vi "Select XNET Signals UI.vi"(8 "error in (no error)":errorcluster, 9 "XNET Cluster":refnum<k21>, 10 "XNET Database":refnum<k21>, 11 "Node Ptr":u64 format="%.0x") -> (0 "error out":errorcluster, 2 "Cancel Out":bool, 3 "XNET Signal Names":refnum<k21>[](array[refnum]))   [LabVIEW 2023, in "J1939 Addon System Explorer.lvlib"]
uses:
  J1939 Addon System Explorer.lvlib
  <vilib>/Utility/cursorutil.llb/Set Cursor (Icon Pict).vi
  Addon Shared/J1939 Addon Shared.lvlib
panel:
  in  "Info?":bool
  in  "Cancel":bool
  in  "Select":bool
  in  "Tree":string(tree)
  # "OUTPUTS"
  # "INPUTS"
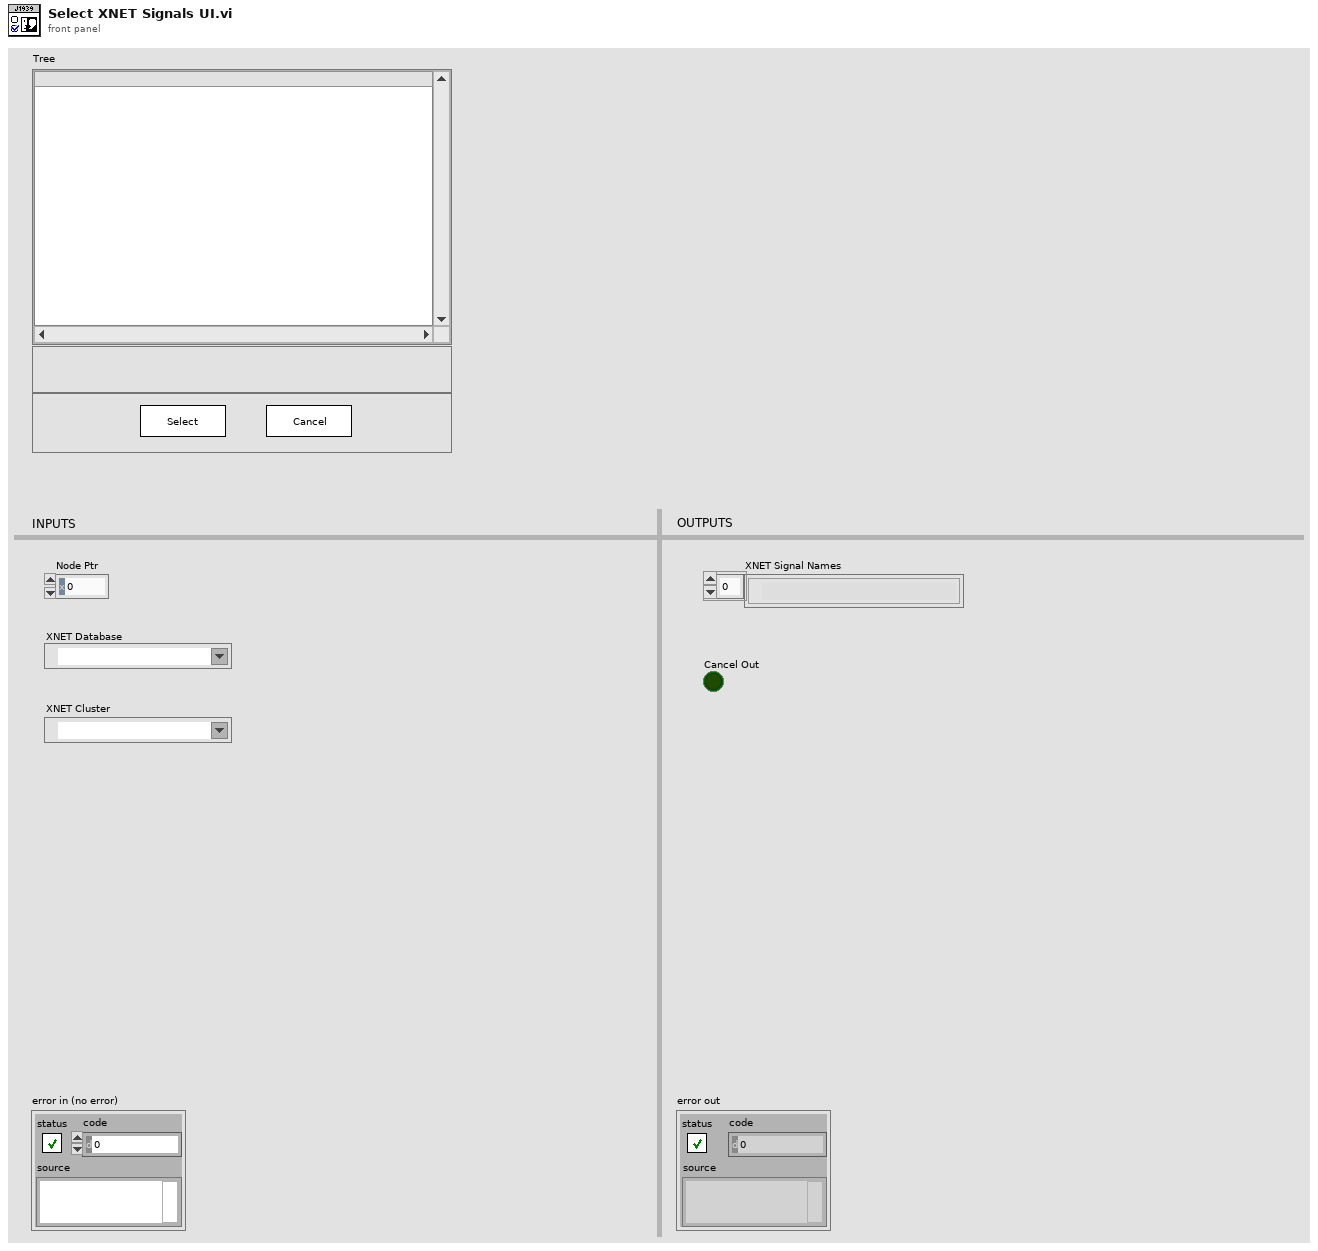
[diagram p1: front panel]
types:
  T1 = typedef "LVPoint32TypeDef.ctl" = cluster{"Horizontal":i32, "Vertical":i32}
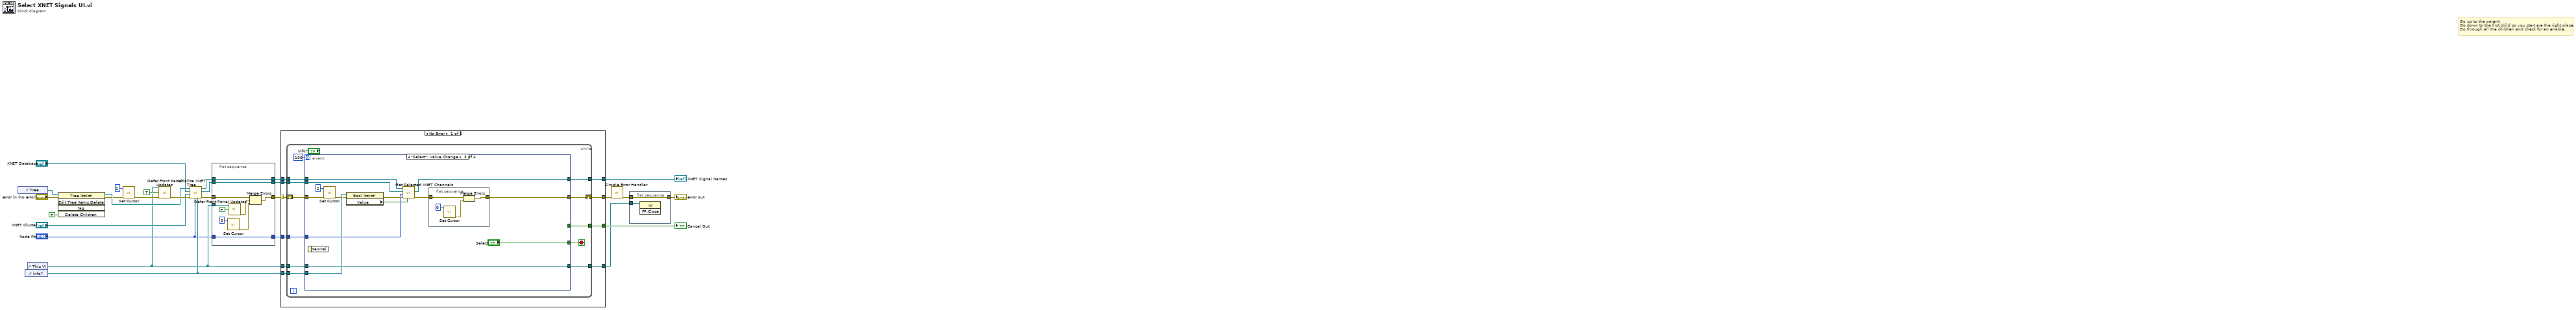
[diagram p0: block diagram]
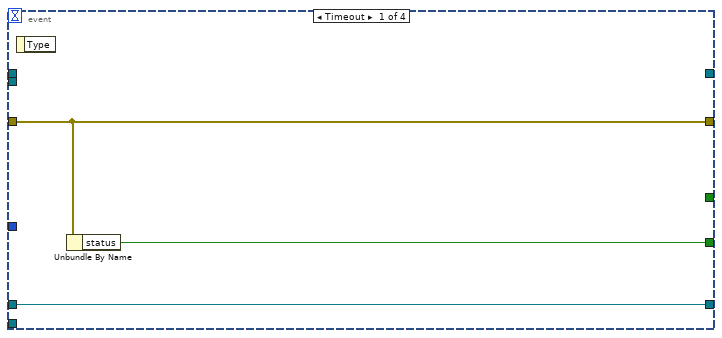
[diagram p2: hidden frame]
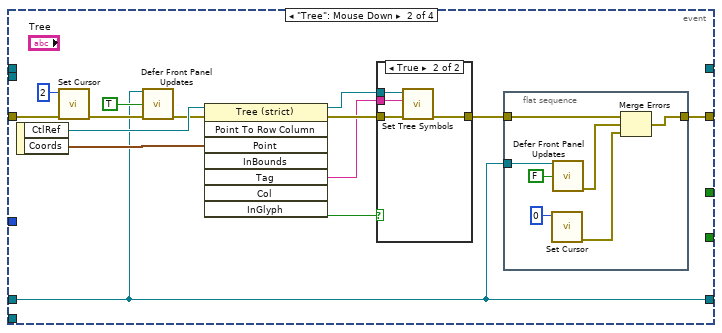
[diagram p3: hidden frame]
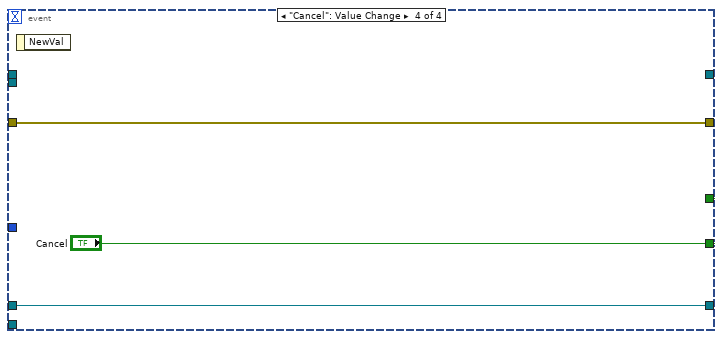
[diagram p5: hidden frame]
diagram:
  # "Go up to the parent.\nGo down to the first child so you start are the right place.\nGo through all the children and check for an enable."
  n1 = control-ref of="Tree"() -> (w14:refnum<vi>)
  n2 = control-ref of="Info?"() -> (w4:refnum<vi>)
  n3 = control-ref of="This VI"() -> (w7:refnum<vi>)
  n4 = invoke on="Invoke Node" class="Tree (strict)" method="Edit Tree Items.Delete"(reference=w14, error in="error in (no error)", "Delete Children"=TRUE ("Delete Children?")) -> (reference out=w13:refnum<vi>, error out=w11:errorcluster)  [unwired: 2 in, 3 out]
  n5 = call-poly <vilib>:"Set Cursor.vi"("error in (no error)"=w11, "icon"=u16 2) -> ("error out"=w10:errorcluster)  [unwired: 8 in, 1 out]
  n6 = call "Defer Front Panel Updates.vi"("This VI"=w7, "Defer Panel Updates"=TRUE, "error in (no error)"=w10) -> ("error out"=w5:errorcluster)  [unwired: 12 in]
  n7 = call "Initialize XNET Tree.vi"("Info?"=w4, "Node Ptr"="Node Ptr", "error in"=w5, "XNET Cluster"="XNET Cluster", "XNET Database"="XNET Database", "Tree"=w13) -> ("error out"=w3:errorcluster, "XNET Cluster Out"=w18:refnum<k21>, "Tree Out"=w1:refnum<vi>)  [unwired: 2 in, 1 out]
  n8 = flat-sequence {
    tunnel: [w36] -> w23
    tunnel: [w33] -> w22
    tunnel: [w31] -> w19
    tunnel: [w30] -> w8
    tunnel: w3 -> [w35]
    tunnel: w1 -> [w33]
    tunnel: w7 -> [w32]
    tunnel: w18 -> [w31]
    tunnel: "Node Ptr" -> [w30]
    frame #0 {
      n9 = call-poly <vilib>:"Set Cursor.vi"("icon"=u16 0) -> ("error out"=w28:errorcluster)  [unwired: 9 in, 1 out]
      n10 = call "Defer Front Panel Updates.vi"("This VI"=w32, "Defer Panel Updates"=FALSE) -> ("error out"=w34:errorcluster)  [unwired: 13 in]
      n11 = Merge Errors(w35, w34, w28) -> (w36:errorcluster)
    }
  }
  n12 = case shown="No Error" w23 {
    selector: w23 -> [w43 w111]
    tunnel: [w47 w111] -> w17
    tunnel: [w46 _] -> w27
    tunnel: [w45 _] -> w26
    tunnel: w8 -> [w44 _]
    tunnel: w22 -> [w42 _]
    tunnel: w19 -> [w41 _]
    tunnel: w7 -> [w40 w110]
    tunnel: [w39 w110] -> w6
    tunnel: w4 -> [w38 _]
    frame No Error {
      n13 = while {
        shift-right: [w57] -> w47
        shift-left: w43 -> [w59]
        tunnel: w41 -> [w56]
        tunnel: [w55] -> w46
        tunnel: [w54] -> w45
        tunnel: w44 -> [w53]
        tunnel: w42 -> [w52]
        tunnel: w40 -> [w50]
        tunnel: [w49] -> w39
        tunnel: w38 -> [w48]
        stop <- w58 stop-if-true
        n14 = event shown="[2] \"Select\": Value Change" {
          selector: _ -> [_ _ _ _]
          dyn-events: _ -> [_ _ _ _]
          timeout: 100 -> [_ _ _ _]
          tunnel: w59 -> [w62 w69 w96 w109]
          tunnel: [w61 _ "Select" "Cancel"] -> w58
          tunnel: [w62 w67 w95 w109] -> w57
          tunnel: w56 -> [_ _ w101 _]
          tunnel: [_ _ w100 _] -> w55
          tunnel: [_ _ _ "Cancel"] -> w54
          tunnel: w53 -> [_ _ w99 _]
          tunnel: w52 -> [_ _ w98 _]
          tunnel: w50 -> [w60 w63 w93 w107]
          tunnel: [w60 w63 w93 w107] -> w49
          tunnel: w48 -> [_ _ w92 _]
          event Timeout {
            n15 = event-data() -> ()  [unwired: 1 in, 1 out]
            n16 = Unbundle By Name(w62) -> ("status"=w61:bool)
          }
          event "Tree": Mouse Down {
            n17 = event-data() -> ("CtlRef"=w75:refnum<vi>, "Coords"=w76:T1)  [unwired: 1 in]
            n18 = call-poly <vilib>:"Set Cursor.vi"("error in (no error)"=w69, "icon"=u16 2) -> ("error out"=w65:errorcluster)  [unwired: 8 in, 1 out]
            n19 = call "Defer Front Panel Updates.vi"("This VI"=w63, "Defer Panel Updates"=TRUE, "error in (no error)"=w65) -> ("error out"=w64:errorcluster)  [unwired: 12 in]
            n20 = invoke on="Invoke Node" class="Tree (strict)" method="Point To Row Column"(reference=w75, error in=w64, "Point"=w76) -> (reference out=w73:refnum<vi>, error out=w74:errorcluster, "Tag"=w72:string, "InGlyph"=w71:bool)  [unwired: 5 in, 4 out]
            n21 = case shown="True" w71 {
              tunnel: w74 -> [w84 w88]
              tunnel: w73 -> [_ w87]
              tunnel: w72 -> [_ w86]
              tunnel: [w84 w85] -> w68
              frame False {
              }
              frame True {
                n22 = call "Set Tree Symbols.vi"("error in"=w88, "Tag"=w86, "CtlRef"=w87) -> ("error out"=w85:errorcluster)  [unwired: 8 in]
              }
            }
            n23 = flat-sequence {
              tunnel: [w80] -> w67
              tunnel: w68 -> [w81]
              tunnel: w63 -> [w77]
              frame #0 {
                n24 = call-poly <vilib>:"Set Cursor.vi"("icon"=u16 0) -> ("error out"=w82:errorcluster)  [unwired: 9 in, 1 out]
                n25 = call "Defer Front Panel Updates.vi"("This VI"=w77, "Defer Panel Updates"=FALSE) -> ("error out"=w78:errorcluster)  [unwired: 13 in]
                n26 = Merge Errors(w81, w78, w82) -> (w80:errorcluster)
              }
            }
          }
          event "Select": Value Change {
            n27 = event-data() -> ()  [unwired: 1 in, 1 out]
            n28 = call-poly <vilib>:"Set Cursor.vi"("error in (no error)"=w96, "icon"=u16 2) -> ("error out"=w91:errorcluster)  [unwired: 8 in, 1 out]
            n29 = property class="Bool (strict)"(reference=w92, error in=w91) -> (error out=w90:errorcluster, "Value"=w89:bool)  [unwired: 1 out]
            n30 = call "Get Selected XNET Channels.vi"("Add Info?"=w89, "error in (no error)"=w90, "Node Ptr"=w99, "XNET Cluster"=w101, "Tree In"=w98) -> ("error out"=w94:errorcluster, "XNET Signal Names"=w100:refnum<k21>[])  [unwired: 4 in, 1 out]
            n31 = flat-sequence {
              tunnel: [w103] -> w95
              tunnel: w94 -> [w104]
              frame #0 {
                n32 = call-poly <vilib>:"Set Cursor.vi"("icon"=u16 0) -> ("error out"=w105:errorcluster)  [unwired: 9 in, 1 out]
                n33 = Merge Errors(w104, w105) -> (w103:errorcluster)
              }
            }
          }
          event "Cancel": Value Change {
            n34 = event-data() -> ()  [unwired: 1 in, 1 out]
          }
        }
      }
    }
    frame Error {
    }
  }
  "XNET Signal Names" <- w27
  "Cancel Out" <- w26
  n35 = call <vilib>:"Simple Error Handler.vi"("error in (no error)"=w17) -> ("error out"=w16:errorcluster)  [unwired: 4 in, 4 out]
  n36 = flat-sequence {
    tunnel: [w113] -> w24
    tunnel: w16 -> [w113]
    tunnel: w6 -> [w112]
    frame #0 {
      n37 = invoke class="VI" method="FP.Close"(reference=w112) -> ()  [unwired: 2 in, 3 out]
    }
  }
  "error out" <- w24
